vi "TimeForTicklish.vi"(4 "time":dbl) -> (1 "String":string)   [LabVIEW 2015]
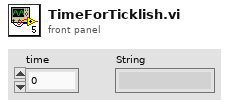
[diagram p1: front panel]
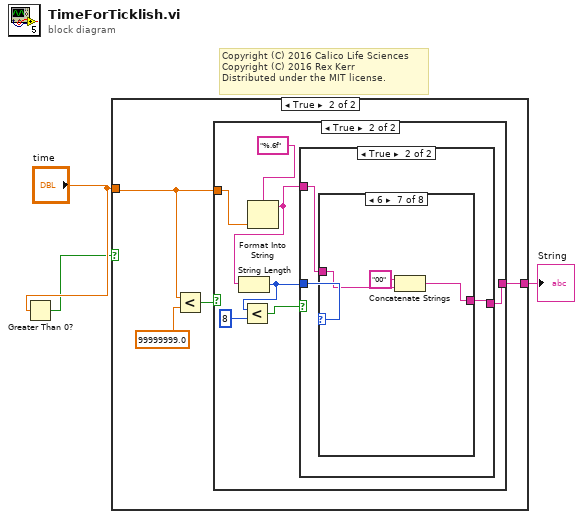
[diagram p0: block diagram]
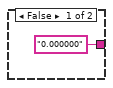
[diagram p2: hidden frame]
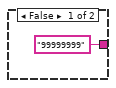
[diagram p3: hidden frame]
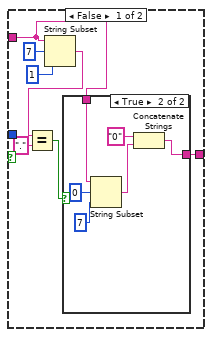
[diagram p4: hidden frame]
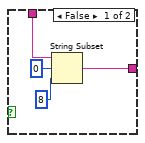
[diagram p5: hidden frame]
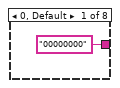
[diagram p6: hidden frame]
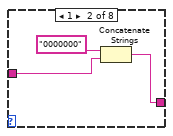
[diagram p7: hidden frame]
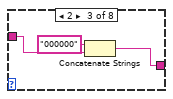
[diagram p8: hidden frame]
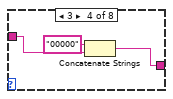
[diagram p9: hidden frame]
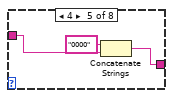
[diagram p10: hidden frame]
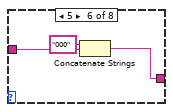
[diagram p11: hidden frame]
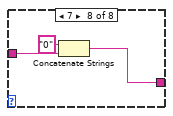
[diagram p12: hidden frame]
diagram:
  # "Copyright (C) 2016 Calico Life Sciences\nCopyright (C) 2016 Rex Kerr\nDistributed under the MIT license."
  n1 = Greater Than 0?(x="time") -> (x > 0?=w2:bool)
  n2 = case shown="True" w2 {
    tunnel: "time" -> [_ w7]
    tunnel: ["0.000000" w5] -> w1
    frame False {
    }
    frame True {
      n3 = Less?(x=w7, y=99999999.0) -> (x < y?=w8:bool)
      n4 = case shown="True" w8 {
        tunnel: w7 -> [_ w16]
        tunnel: ["99999999" w11] -> w5
        frame False {
        }
        frame True {
          n5 = Format Into String(format string="%.6f" ("initial string"), w16) -> (resulting string=w13:string)  [unwired: 2 in, 1 out]
          n6 = String Length(string=w13) -> (length=w12:i32)
          n7 = Less?(x=w12, y=8) -> (x < y?=w14:bool)
          n8 = case shown="True" w14 {
            tunnel: w13 -> [w18 w35]
            tunnel: [w17 w34] -> w11
            tunnel: w12 -> [_ w36]
            frame False {
              n9 = String Subset(string=w18, offset (0)=7, length (rest)=1 ("length (rest)")) -> (substring=w21:string)
              n10 = Equal?(x=w21, y=".") -> (x = y?=w19:bool)
              n11 = case shown="True" w19 {
                tunnel: w18 -> [w27 w33]
                tunnel: [w24 w32] -> w17
                frame False {
                  n12 = String Subset(string=w27, offset (0)=0, length (rest)=8 ("length (rest)")) -> (substring=w24:string)
                }
                frame True {
                  n13 = String Subset(string=w33, offset (0)=0, length (rest)=7 ("length (rest)")) -> (substring=w30:string)
                  n14 = Concatenate Strings("0" ("string"), w30) -> (w32:string)
                }
              }
            }
            frame True {
              n15 = case shown="6" w36 {
                tunnel: w35 -> [_ w39 w42 w45 w48 w51 w54 w58]
                tunnel: ["00000000" w38 w41 w44 w47 w50 w53 w56] -> w34
                frame 0, Default {
                }
                frame 1 {
                  n16 = Concatenate Strings("0000000" ("string"), w39) -> (w38:string)
                }
                frame 2 {
                  n17 = Concatenate Strings("000000" ("string"), w42) -> (w41:string)
                }
                frame 3 {
                  n18 = Concatenate Strings("00000" ("string"), w45) -> (w44:string)
                }
                frame 4 {
                  n19 = Concatenate Strings("0000" ("string"), w48) -> (w47:string)
                }
                frame 5 {
                  n20 = Concatenate Strings("000" ("string"), w51) -> (w50:string)
                }
                frame 6 {
                  n21 = Concatenate Strings("00" ("string"), w54) -> (w53:string)
                }
                frame 7 {
                  n22 = Concatenate Strings("0" ("string"), w58) -> (w56:string)
                }
              }
            }
          }
        }
      }
    }
  }
  "String" <- w1
